vi "Magazine_Set.vi"   [LabVIEW 2019]
uses:
  Magazine_States.ctl
  Globals/Magazine_Globals.vi
  Globals/Sensor_Values.vi
types:
  T1 = typedef "Magazine_States.ctl" = enum16{"No-Op", "Loading", "Fire", "Unjam", "Manual_Percent_Voltage", "Manual_Speed_Control"}
  T2 = typedef "Magazine_Cluster.ctl" = cluster{"Fire":bool, "Magazine_Throttle":dbl, "Control_States":T1}
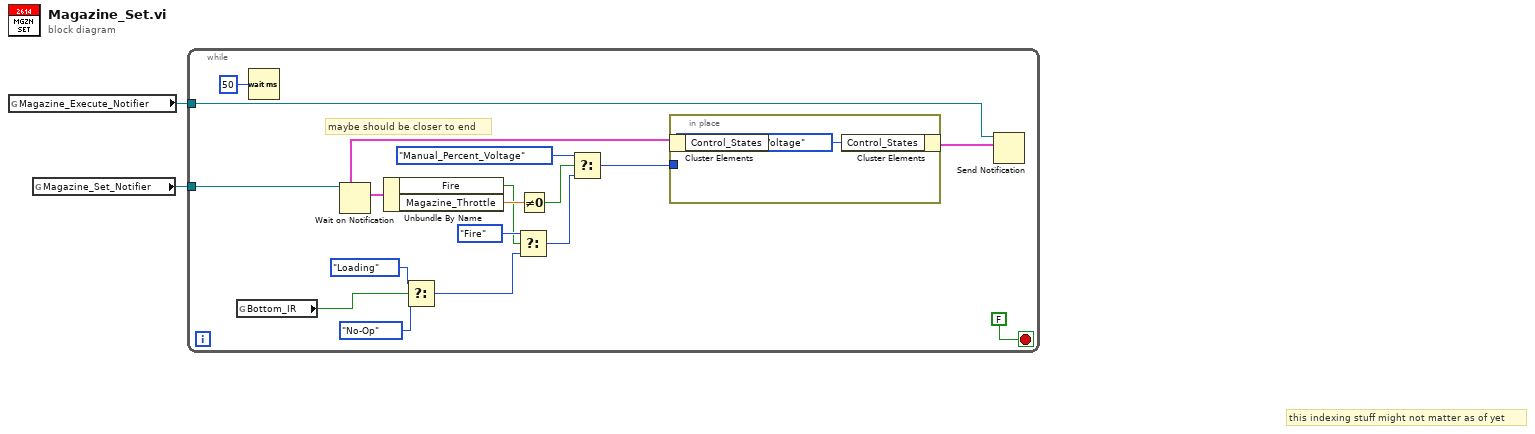
[diagram p0: block diagram]
diagram:
  # "this indexing stuff might not matter as of yet"
  n1 = global read "Magazine_Globals.vi" "Magazine_Execute_Notifier"() -> (w1:refnum<notifier>)
  n2 = global read "Magazine_Globals.vi" "Magazine_Set_Notifier"() -> (w2:refnum<notifier>)
  n3 = while {
    tunnel: w2 -> [w18]
    tunnel: w1 -> [w17]
    stop <- FALSE stop-if-true
    # "maybe should be closer to end"
    n4 = global read "Sensor_Values.vi" "Bottom_IR"() -> (w7:bool)
    n5 = Wait (ms)(milliseconds to wait=u32 50) -> ()  [unwired: 1 out]
    n6 = Wait on Notification(notifier=w18) -> (notification=w15:T2)  [unwired: 3 in, 3 out]
    n7 = Unbundle By Name(w15) -> ("Fire"=w3:bool, "Magazine_Throttle"=w12:dbl)
    n8 = Select(t=Magazine_States."Loading" ("f"), s=w7, f=Magazine_States."No-Op" ("Control_States")) -> (s? t:f=w8:T1)
    n9 = Select(t=Magazine_States."Fire" ("f"), s=w3, f=w8) -> (s? t:f=w11:T1)
    n10 = Not Equal To 0?(x=w12) -> (x != 0?=w14:bool)
    n11 = Select(t=Magazine_States."Manual_Percent_Voltage", s=w14, f=w11) -> (s? t:f=w6:T1)
    n12 = in-place {
      in-place-border: w6 -> [_]
      n13 = in-place-cluster #1(w15) -> ()  [unwired: 1 out]
      n14 = in-place-cluster #1("Control_States"=Magazine_States."Manual_Percent_Voltage") -> (w16:T2)
    }
    n15 = Send Notification(notification=w16, notifier=w17) -> ()  [unwired: 1 in, 2 out]
  }
